vi "Tims Tools - 2D Array Multi Column Sort with Ascending Descending Selection SGL.vi"(2 "Priority Columns (0)":i32[](array[numeric]), 7 "Ascending and Descending Sample Data":sgl[][](array[numeric]), 13 "Descending (F)":bool) -> (8 "Sorted Data":sgl[][](array[numeric]))   [LabVIEW 2018]
doc: "<B>2D Array Multi Column Sort with Ascending Descending Selection</B>\n\nTakes one or more sort column requests and processes all rows into Ascending or Descending sort order based on the user's selection.\n\nNOTE: This algorithm is based on the example provided by a. h. on NI's website (https://decibel.ni.com/content/people/a.h.). This update:\n\n- Corrects an incorrect placement of Invert Array that caused errors in secondary columns of a multi-column sort when Descending = True\n- Adds protection against having too many search elements in the Priority Columns input\n- Documents the solution\n<B>\nTim Jones\n9/28/2016"
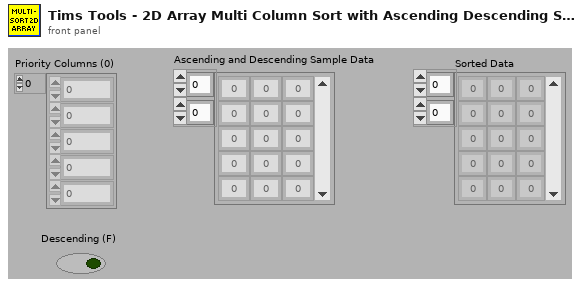
[diagram p1: front panel]
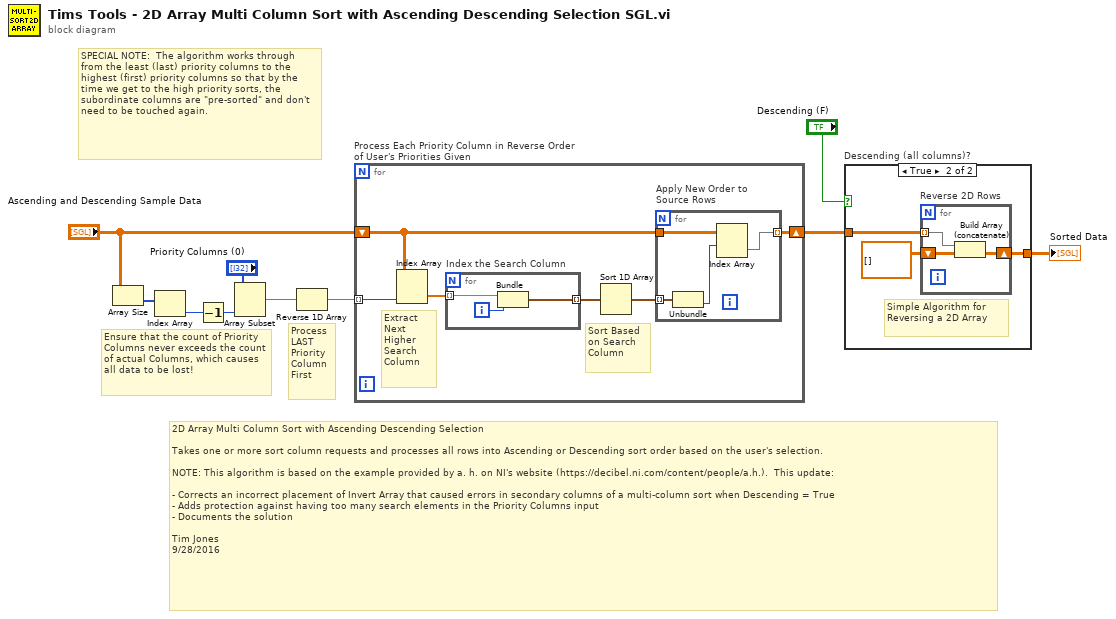
[diagram p0: block diagram]
diagram:
  # "2D Array Multi Column Sort with Ascending Descending Selection\n\nTakes one or more sort column requests and processes all rows into Ascending or Descending sort order based on the user's selection.\n\nNOTE: This algorithm is based on the example provided by a. h. on NI's website (https://decibel.ni.com/content/people/a.h.).  This update:\n\n- Corrects an incorrect placement of Invert Array that caused errors in secondary columns of a multi-column sort when Descending = True\n- Adds protection against having too many search elements in the Priority Columns input\n- Documents the solution\n\nTim Jones\n9/28/2016"
  # "Ensure that the count of Priority Columns never exceeds the count of actual Columns, which causes all data to be lost!"
  # "SPECIAL NOTE:  The algorithm works through from the least (last) priority columns to the highest (first) priority columns so that by the time we get to the high priority sorts, the subordinate columns are \"pre-sorted\" and don't need to be touched again."
  # "Process\nLAST\nPriority\nColumn\nFirst"
  n1 = Array Size(array="Ascending and Descending Sample Data") -> (size(s)=w6:i32[])
  n2 = Index Array(array=w6) -> (element=w5:i32)  [unwired: 1 in]
  n3 = Decrement(x=w5) -> (x-1=w1:i32)
  n4 = Array Subset(array="Priority Columns (0)", length=w1) -> (w3:i32[])  [unwired: 1 in]
  n5 = Reverse 1D Array(array=w3) -> (reversed array=w10:i32[])
  n6 = for "Process Each Priority Column in Reverse Order of User's Priorities Given" {
    shift-right: [w12] -> w9
    shift-left: "Ascending and Descending Sample Data" -> [w11]
    tunnel: w10 -> [w14] mode=indexing
    # "Sort Based on Search Column"
    # "Extract Next Higher Search Column"
    n7 = Index Array(array=w11, index (col)=w14) -> (element=w16:sgl[])  [unwired: 1 in]
    n8 = for "Index the Search Column" {
      tunnel: w16 -> [w21] mode=indexing
      tunnel: [w23] -> w15 mode=indexing
      i -> [w22]
      n9 = Bundle("number: 0 to 1"=w21, w22) -> (w23:cluster{"number: 0 to 1":sgl, i32})  [unwired: 1 out]
    }
    n10 = Sort 1D Array(array=w15) -> (sorted array=w13:cluster{"number: 0 to 1":sgl, i32}[])
    n11 = for "Apply New Order to Source Rows" {
      tunnel: w13 -> [w20] mode=indexing
      tunnel: w11 -> [w18]
      tunnel: [w19] -> w12 mode=indexing
      n12 = Unbundle(w20) -> (w17:i32)  [unwired: 1 out]
      n13 = Index Array(array=w18, index (row)=w17) -> (element=w19:sgl[])  [unwired: 1 in]
    }
  }
  n14 = case "Descending (all columns)?" shown="True" "Descending (F)" {
    tunnel: w9 -> [w24 w26]
    tunnel: [w24 w25] -> w8
    frame False {
    }
    frame True {
      # "Simple Algorithm for Reversing a 2D Array"
      n15 = for "Reverse 2D Rows" {
        tunnel: w26 -> [w30] mode=indexing
        shift-right: [w28] -> w25
        shift-left: sgl[][] [] -> [w29]
        n16 = Build Array (concatenate)(w30, w29) -> (w28:sgl[][])
      }
    }
  }
  "Sorted Data" <- w8
